vi "test Create New Import Status Channels.vi"(8 "error in (no error)":errorcluster, 11 "TestCase in":refnum<class "Routing and Faulting Import Unit Tests.lvclass">) -> (0 "error out":errorcluster, 3 "TestCase out":refnum<class "Routing and Faulting Import Unit Tests.lvclass">)   [LabVIEW 2020, in "Routing and Faulting Import Unit Tests.lvclass"]
uses:
  Routing and Faulting Import Unit Tests.lvclass
  <vilib>/NI VeriStand/Custom Device API/Custom Device Channel.ctl
  <vilib>/NI VeriStand/Custom Device API/Custom Device Channel Type.ctl
  <vilib>/addons/_JKI Toolkits/VI Tester/TestCase.llb/TestCase.lvclass
  <vilib>/NI VeriStand/Custom Device Tools/Custom Device Utility Library/Custom Device Utility Library.lvlib
  <vilib>/NI VeriStand/Custom Device API/Custom Device API.lvlib
  C:/Program Files (x86)/National Instruments/LabVIEW 2020/vi.lib/addons/_JKI Toolkits/VI Tester/TestCase.llb/TestCase.lvclass
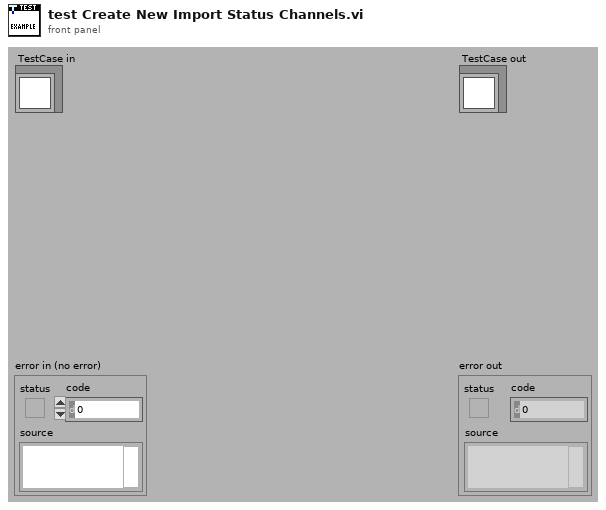
[diagram p1: front panel]
types:
  T1 = typedef "Custom Device API.lvlib/Custom Device Channel.ctl" = cluster{"Type":T2, "Units":string, "Default Value":dbl, "Faultable":bool, "Scalable":bool}
  T2 = typedef "Custom Device API.lvlib/Custom Device Channel Type.ctl" = enum16{"Input", "Output"}
  T3 = typedef "Custom Device API.lvlib/Custom Device Item Ref.ctl" = u64
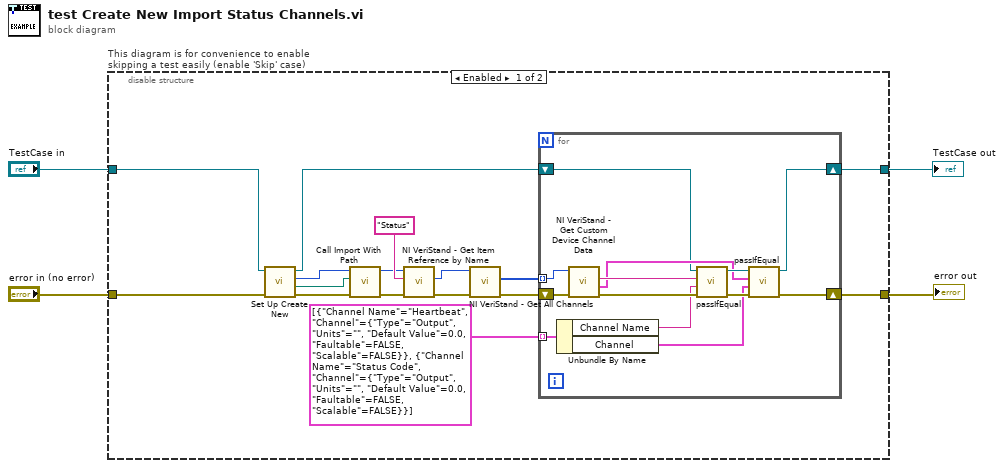
[diagram p0: block diagram]
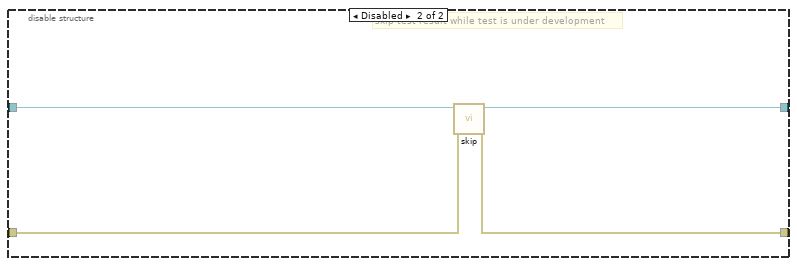
[diagram p2: hidden frame]
diagram:
  n1 = disable-structure "This diagram is for convenience to enable skipping a test easily (enable 'Skip' case)" shown="Enabled" {
    disable-tunnel: "TestCase in" -> [w18 w37]
    disable-tunnel: [w8 w35] -> w1
    disable-tunnel: [w11 w36] -> w3
    disable-tunnel: "error in (no error)" -> [w19 w34]
    frame Enabled {
      n2 = call "Set Up Create New.vi"("error in (no error)"=w19, "Test Case in"=w18) -> ("error out"=w20:errorcluster, "Import Path"=w7:path, "Routing and Faulting Custom Device Ref"=w6:T3, "Test Case out"=w9:refnum<class "Routing and Faulting Import Unit Tests.lvclass">)  [unwired: 6 in]
      n3 = call "Call Import With Path.vi"("error in (no error)"=w20, "Path"=w7, "Routing and Faulting Custom Device Ref in"=w6) -> ("error out"=w17:errorcluster, "Routing and Faulting Custom Device Ref out"=w5:T3)  [unwired: 7 in]
      n4 = call <vilib>:"NI VeriStand - Get Item Reference by Name.vi"("error in (no error)"=w17, "Item Name"="Status", "Parent Ref in"=w5) -> ("error out"=w15:errorcluster, "Item Ref"=w14:T3)  [unwired: 5 in, 2 out]
      n5 = call <vilib>:"NI VeriStand - Get All Channels.vi"("error in"=w15, "Section Ref in"=w14) -> ("error out"=w13:errorcluster, "Channel Refs"=w12:T3[])  [unwired: 6 in, 2 out]
      n6 = for {
        shift-right: [w23] -> w11
        shift-left: w13 -> [w33]
        tunnel: w12 -> [w32] mode=indexing
        tunnel: cluster{"Channel Name":string, "Channel":T1}[] [{"Channel Name"="Heartbeat", "Channel"={"Type"=enum."Output", "Units"="", "Default Value"=0.0, "Faultable"=FALSE, "Scalable"=FALSE}}, {"Channel Name"="Status Code", "Channel"={"Type"=enum."Output", "Units"="", "Default Value"=0.0, "Faultable"=FALSE, "Scalable"=FALSE}}] -> [w31] mode=indexing
        shift-right: [w21] -> w8
        shift-left: w9 -> [w22]
        n7 = Unbundle By Name(w31) -> ("Channel Name"=w26:string, "Channel"=w24:T1)
        n8 = call <vilib>:"NI VeriStand - Get Custom Device Channel Data.vi"("error in (no error)"=w33, "Channel Ref in"=w32) -> ("error out"=w30:errorcluster, "Channel"=w25:T1, "Channel Name"=w27:string)  [unwired: 4 in, 3 out]
        n9 = call-dynamic "passIfEqual.vi"("error in (no error)"=w30, "y"=w26, "x"=w27, "TestCase in"=w22) -> ("error out"=w29:errorcluster, "TestCase out"=w28:refnum<class "Routing and Faulting Import Unit Tests.lvclass">)  [unwired: 6 in]
        n10 = call-dynamic "passIfEqual.vi"("error in (no error)"=w29, "y"=w24, "x"=w25, "TestCase in"=w28) -> ("error out"=w23:errorcluster, "TestCase out"=w21:refnum<class "Routing and Faulting Import Unit Tests.lvclass">)  [unwired: 6 in]
      }
    }
    frame Disabled {
      # "skip test result while test is under development"
      n11 = call <vilib>:"skip.vi"("error in (no error)"=w34, "TestCase in"=w37) -> ("error out"=w36:errorcluster, "TestCase out"=w35:refnum<class "Routing and Faulting Import Unit Tests.lvclass">)  [unwired: 8 in]
    }
  }
  "error out" <- w3
  "TestCase out" <- w1
